vi "Test - Draw Teapot.vi"() -> ()   [LabVIEW 2022 SP3, in "Raster.lvlib"] (continued)
"y"=370.30228, "z"=0.9852259}, "UV"={"u"=0.0, "v"=0.0}, "Colour"=12517256}, "Vertex 3"={"Position"={"x"=479.53958, "y"=369.04208, "z"=0.98549163}, "UV"={"u"=0.0, "v"=0.0}, "Colour"=12517256}, "Alpha"=0.0, "Alpha Blending Enabled"=FALSE, "Colour"=11463293}, {"Vertex 1"={"Position"={"x"=221.22188, "y"=231.18608, "z"=0.9853604}, "UV"={"u"=0.0, "v"=0.0}, "Colour"=12517256}, "Vertex 2"={"Position"={"x"=225.54918, "y"=253.65358, "z"=0.9854739}, "UV"={"u"=0.0, "v"=0.0}, "Colour"=12517256}, "Vertex 3"={"Position"={"x"=257.52774, "y"=251.44232, "z"=0.9847784}, "UV"={"u"=0.0, "v"=0.0}, "Colour"=12517256}, "Alpha"=0.0, "Alpha Blending Enabled"=FALSE, "Colour"=9289317}, {"Vertex 1"={"Position"={"x"=479.53958, "y"=369.04208, "z"=0.98549163}, "UV"={"u"=0.0, "v"=0.0}, "Colour"=12517256}, "Vertex 2"={"Position"={"x"=484.57294, "y"=346.33105, "z"=0.98520327}, "UV"={"u"=0.0, "v"=0.0}, "Colour"=12517256}, "Vertex 3"={"Position"={"x"=444.34033, "y"=347.23126, "z"=0.9849148}, "UV"={"u"=0.0, "v"=0.0}, "Colour"=12517256}, "Alpha"=0.0, "Alpha Blending Enabled"=FALSE, "Colour"=11463293}, {"Vertex 1"={"Position"={"x"=486.9139, "y"=106.21548, "z"=0.98506916}, "UV"={"u"=0.0, "v"=0.0}, "Colour"=12517256}, "Vertex 2"={"Position"={"x"=481.5222, "y"=99.90905, "z"=0.985378}, "UV"={"u"=0.0, "v"=0.0}, "Colour"=12517256}, "Vertex 3"={"Position"={"x"=442.71094, "y"=96.16424, "z"=0.9851035}, "UV"={"u"=0.0, "v"=0.0}, "Colour"=12517256}, "Alpha"=0.0, "Alpha Blending Enabled"=FALSE, "Colour"=131841}, {"Vertex 1"={"Position"={"x"=315.42706, "y"=346.33105, "z"=0.98520327}, "UV"={"u"=0.0, "v"=0.0}, "Colour"=12517256}, "Vertex 2"={"Position"={"x"=310.53198, "y"=322.8849, "z"=0.98492277}, "UV"={"u"=0.0, "v"=0.0}, "Colour"=12517256}, "Vertex 3"={"Position"={"x"=274.2394, "y"=322.16803, "z"=0.9853966}, "UV"={"u"=0.0, "v"=0.0}, "Colour"=12517256}, "Alpha"=0.0, "Alpha Blending Enabled"=FALSE, "Colour"=11001975}, {"Vertex 1"={"Position"={"x"=277.72037, "y"=112.11777, "z"=0.98552537}, "UV"={"u"=0.0, "v"=0.0}, "Colour"=12517256}, "Vertex 2"={"Position"={"x"=270.06448, "y"=120.58319, "z"=0.98524225}, "UV"={"u"=0.0, "v"=0.0}, "Colour"=12517256}, "Vertex 3"={"Position"={"x"=307.46243, "y"=114.58211, "z"=0.98474693}, "UV"={"u"=0.0, "v"=0.0}, "Colour"=12517256}, "Alpha"=0.0, "Alpha Blending Enabled"=FALSE, "Colour"=131841}, {"Vertex 1"={"Position"={"x"=359.82788, "y"=91.52895, "z"=0.98539746}, "UV"={"u"=0.0, "v"=0.0}, "Colour"=12517256}, "Vertex 2"={"Position"={"x"=357.28906, "y"=96.16424, "z"=0.9851035}, "UV"={"u"=0.0, "v"=0.0}, "Colour"=12517256}, "Vertex 3"={"Position"={"x"=400.0, "y"=94.84046, "z"=0.9850064}, "UV"={"u"=0.0, "v"=0.0}, "Colour"=12517256}, "Alpha"=0.0, "Alpha Blending Enabled"=FALSE, "Colour"=131841}, {"Vertex 1"={"Position"={"x"=580.64856, "y"=168.66481, "z"=0.9853113}, "UV"={"u"=0.0, "v"=0.0}, "Colour"=12517256}, "Vertex 2"={"Position"={"x"=575.6004, "y"=152.34836, "z"=0.9854437}, "UV"={"u"=0.0, "v"=0.0}, "Colour"=12517256}, "Vertex 3"={"Position"={"x"=543.45624, "y"=145.25499, "z"=0.98474205}, "UV"={"u"=0.0, "v"=0.0}, "Colour"=12517256}, "Alpha"=0.0, "Alpha Blending Enabled"=FALSE, "Colour"=4413744}, {"Vertex 1"={"Position"={"x"=267.97037, "y"=298.8649, "z"=0.98516476}, "UV"={"u"=0.0, "v"=0.0}, "Colour"=12517256}, "Vertex 2"={"Position"={"x"=274.2394, "y"=322.16803, "z"=0.9853966}, "UV"={"u"=0.0, "v"=0.0}, "Colour"=12517256}, "Vertex 3"={"Position"={"x"=310.53198, "y"=322.8849, "z"=0.98492277}, "UV"={"u"=0.0, "v"=0.0}, "Colour"=12517256}, "Alpha"=0.0, "Alpha Blending Enabled"=FALSE, "Colour"=10804598}, {"Vertex 1"={"Position"={"x"=574.4508, "y"=253.65358, "z"=0.9854739}, "UV"={"u"=0.0, "v"=0.0}, "Colour"=12517256}, "Vertex 2"={"Position"={"x"=578.77814, "y"=231.18608, "z"=0.9853604}, "UV"={"u"=0.0, "v"=0.0}, "Colour"=12517256}, "Vertex 3"={"Position"={"x"=546.1793, "y"=227.81743, "z"=0.98464125}, "UV"={"u"=0.0, "v"=0.0}, "Colour"=12517256}, "Alpha"=0.0, "Alpha Blending Enabled"=FALSE, "Colour"=9289317}, {"Vertex 1"={"Position"={"x"=400.0, "y"=90.25612, "z"=0.985308}, "UV"={"u"=0.0, "v"=0.0}, "Colour"=12517256}, "Vertex 2"={"Position"={"x"=400.0, "y"=94.84046, "z"=0.9850064}, "UV"={"u"=0.0, "v"=0.0}, "Colour"=12517256}, "Vertex 3"={"Position"={"x"=442.71094, "y"=96.16424, "z"=0.9851035}, "UV"={"u"=0.0, "v"=0.0}, "Colour"=12517256}, "Alpha"=0.0, "Alpha Blending Enabled"=FALSE, "Colour"=131841}, {"Vertex 1"={"Position"={"x"=542.4723, "y"=251.44232, "z"=0.9847784}, "UV"={"u"=0.0, "v"=0.0}, "Colour"=12517256}, "Vertex 2"={"Position"={"x"=537.67664, "y"=275.21597, "z"=0.9849558}, "UV"={"u"=0.0, "v"=0.0}, "Colour"=12517256}, "Vertex 3"={"Position"={"x"=568.8375, "y"=276.3083, "z"=0.9856211}, "UV"={"u"=0.0, "v"=0.0}, "Colour"=12517256}, "Alpha"=0.0, "Alpha Blending Enabled"=FALSE, "Colour"=9750122}, {"Vertex 1"={"Position"={"x"=256.5438, "y"=145.25499, "z"=0.98474205}, "UV"={"u"=0.0, "v"=0.0}, "Colour"=12517256}, "Vertex 2"={"Position"={"x"=262.76135, "y"=131.49307, "z"=0.984972}, "UV"={"u"=0.0, "v"=0.0}, "Colour"=12517256}, "Vertex 3"={"Position"={"x"=231.67577, "y"=138.89714, "z"=0.98563457}, "UV"={"u"=0.0, "v"=0.0}, "Colour"=12517256}, "Alpha"=0.0, "Alpha Blending Enabled"=FALSE, "Colour"=2371610}, {"Vertex 1"={"Position"={"x"=358.34668, "y"=370.30228, "z"=0.9852259}, "UV"={"u"=0.0, "v"=0.0}, "Colour"=12517256}, "Vertex 2"={"Position"={"x"=355.65967, "y"=347.23126, "z"=0.9849148}, "UV"={"u"=0.0, "v"=0.0}, "Colour"=12517256}, "Vertex 3"={"Position"={"x"=315.42706, "y"=346.33105, "z"=0.98520327}, "UV"={"u"=0.0, "v"=0.0}, "Colour"=12517256}, "Alpha"=0.0, "Alpha Blending Enabled"=FALSE, "Colour"=11463293}, {"Vertex 1"={"Position"={"x"=307.46243, "y"=114.58211, "z"=0.98474693}, "UV"={"u"=0.0, "v"=0.0}, "Colour"=12517256}, "Vertex 2"={"Position"={"x"=313.0861, "y"=106.21548, "z"=0.98506916}, "UV"={"u"=0.0, "v"=0.0}, "Colour"=12517256}, "Vertex 3"={"Position"={"x"=277.72037, "y"=112.11777, "z"=0.98552537}, "UV"={"u"=0.0, "v"=0.0}, "Colour"=12517256}, "Alpha"=0.0, "Alpha Blending Enabled"=FALSE, "Colour"=131841}, {"Vertex 1"={"Position"={"x"=224.39961, "y"=152.34836, "z"=0.9854437}, "UV"={"u"=0.0, "v"=0.0}, "Colour"=12517256}, "Vertex 2"={"Position"={"x"=219.35144, "y"=168.66481, "z"=0.9853113}, "UV"={"u"=0.0, "v"=0.0}, "Colour"=12517256}, "Vertex 3"={"Position"={"x"=252.2155, "y"=162.16495, "z"=0.9845819}, "UV"={"u"=0.0, "v"=0.0}, "Colour"=12517256}, "Alpha"=0.0, "Alpha Blending Enabled"=FALSE, "Colour"=4413744}, {"Vertex 1"={"Position"={"x"=218.445, "y"=209.18083, "z"=0.98528755}, "UV"={"u"=0.0, "v"=0.0}, "Colour"=12517256}, "Vertex 2"={"Position"={"x"=221.22188, "y"=231.18608, "z"=0.9853604}, "UV"={"u"=0.0, "v"=0.0}, "Colour"=12517256}, "Vertex 3"={"Position"={"x"=253.82066, "y"=227.81743, "z"=0.98464125}, "UV"={"u"=0.0, "v"=0.0}, "Colour"=12517256}, "Alpha"=0.0, "Alpha Blending Enabled"=FALSE, "Colour"=8761951}, {"Vertex 1"={"Position"={"x"=355.65967, "y"=347.23126, "z"=0.9849148}, "UV"={"u"=0.0, "v"=0.0}, "Colour"=12517256}, "Vertex 2"={"Position"={"x"=358.34668, "y"=370.30228, "z"=0.9852259}, "UV"={"u"=0.0, "v"=0.0}, "Colour"=12517256}, "Vertex 3"={"Position"={"x"=400.0, "y"=370.74744, "z"=0.98513204}, "UV"={"u"=0.0, "v"=0.0}, "Colour"=12517256}, "Alpha"=0.0, "Alpha Blending Enabled"=FALSE, "Colour"=11660927}, {"Vertex 1"={"Position"={"x"=354.40778, "y"=102.34398, "z"=0.9847698}, "UV"={"u"=0.0, "v"=0.0}, "Colour"=12517256}, "Vertex 2"={"Position"={"x"=357.28906, "y"=96.16424, "z"=0.9851035}, "UV"={"u"=0.0, "v"=0.0}, "Colour"=12517256}, "Vertex 3"={"Position"={"x"=318.4778, "y"=99.90905, "z"=0.985378}, "UV"={"u"=0.0, "v"=0.0}, "Colour"=12517256}, "Alpha"=0.0, "Alpha Blending Enabled"=FALSE, "Colour"=131841}, {"Vertex 1"={"Position"={"x"=525.7606, "y"=322.16803, "z"=0.9853966}, "UV"={"u"=0.0, "v"=0.0}, "Colour"=12517256}, "Vertex 2"={"Position"={"x"=532.0296, "y"=298.8649, "z"=0.98516476}, "UV"={"u"=0.0, "v"=0.0}, "Colour"=12517256}, "Vertex 3"={"Position"={"x"=494.0796, "y"=298.8263, "z"=0.9846586}, "UV"={"u"=0.0, "v"=0.0}, "Colour"=12517256}, "Alpha"=0.0, "Alpha Blending Enabled"=FALSE, "Colour"=10804598}, {"Vertex 1"={"Position"={"x"=318.4778, "y"=99.90905, "z"=0.985378}, "UV"={"u"=0.0, "v"=0.0}, "Colour"=12517256}, "Vertex 2"={"Position"={"x"=313.0861, "y"=106.21548, "z"=0.98506916}, "UV"={"u"=0.0, "v"=0.0}, "Colour"=12517256}, "Vertex 3"={"Position"={"x"=354.40778, "y"=102.34398, "z"=0.9847698}, "UV"={"u"=0.0, "v"=0.0}, "Colour"=12517256}, "Alpha"=0.0, "Alpha Blending Enabled"=FALSE, "Colour"=131841}, {"Vertex 1"={"Position"={"x"=262.32336, "y"=275.21597, "z"=0.9849558}, "UV"={"u"=0.0, "v"=0.0}, "Colour"=12517256}, "Vertex 2"={"Position"={"x"=257.52774, "y"=251.44232, "z"=0.9847784}, "UV"={"u"=0.0, "v"=0.0}, "Colour"=12517256}, "Vertex 3"={"Position"={"x"=225.54918, "y"=253.65358, "z"=0.9854739}, "UV"={"u"=0.0, "v"=0.0}, "Colour"=12517256}, "Alpha"=0.0, "Alpha Blending Enabled"=FALSE, "Colour"=9750122}, {"Vertex 1"={"Position"={"x"=578.77814, "y"=231.18608, "z"=0.9853604}, "UV"={"u"=0.0, "v"=0.0}, "Colour"=12517256}, "Vertex 2"={"Position"={"x"=581.555, "y"=209.18083, "z"=0.98528755}, "UV"={"u"=0.0, "v"=0.0}, "Colour"=12517256}, "Vertex 3"={"Position"={"x"=548.5629, "y"=204.66248, "z"=0.9845531}, "UV"={"u"=0.0, "v"=0.0}, "Colour"=12517256}, "Alpha"=0.0, "Alpha Blending Enabled"=FALSE, "Colour"=8761951}, {"Vertex 1"={"Position"={"x"=400.0, "y"=347.54977, "z"=0.98481274}, "UV"={"u"=0.0, "v"=0.0}, "Colour"=12517256}, "Vertex 2"={"Position"={"x"=400.0, "y"=370.74744, "z"=0.98513204}, "UV"={"u"=0.0, "v"=0.0}, "Colour"=12517256}, "Vertex 3"={"Position"={"x"=441.6533, "y"=370.30228, "z"=0.9852259}, "UV"={"u"=0.0, "v"=0.0}, "Colour"=12517256}, "Alpha"=0.0, "Alpha Blending Enabled"=FALSE, "Colour"=11660927}, {"Vertex 1"={"Position"={"x"=537.23865, "y"=131.49307, "z"=0.984972}, "UV"={"u"=0.0, "v"=0.0}, "Colour"=12517256}, "Vertex 2"={"Position"={"x"=543.45624, "y"=145.25499, "z"=0.98474205}, "UV"={"u"=0.0, "v"=0.0}, "Colour"=12517256}, "Vertex 3"={"Position"={"x"=575.6004, "y"=152.34836, "z"=0.9854437}, "UV"={"u"=0.0, "v"=0.0}, "Colour"=12517256}, "Alpha"=0.0, "Alpha Blending Enabled"=FALSE, "Colour"=2371610}, {"Vertex 1"={"Position"={"x"=582.5317, "y"=187.944, "z"=0.9852619}, "UV"={"u"=0.0, "v"=0.0}, "Colour"=12517256}, "Vertex 2"={"Position"={"x"=580.64856, "y"=168.66481, "z"=0.9853113}, "UV"={"u"=0.0, "v"=0.0}, "Colour"=12517256}, "Vertex 3"={"Position"={"x"=547.78455, "y"=162.16495, "z"=0.9845819}, "UV"={"u"=0.0, "v"=0.0}, "Colour"=12517256}, "Alpha"=0.0, "Alpha Blending Enabled"=FALSE, "Colour"=6522183}, {"Vertex 1"={"Position"={"x"=217.4683, "y"=187.944, "z"=0.9852619}, "UV"={"u"=0.0, "v"=0.0}, "Colour"=12517256}, "Vertex 2"={"Position"={"x"=218.445, "y"=209.18083, "z"=0.98528755}, "UV"={"u"=0.0, "v"=0.0}, "Colour"=12517256}, "Vertex 3"={"Position"={"x"=251.43709, "y"=204.66248, "z"=0.9845531}, "UV"={"u"=0.0, "v"=0.0}, "Colour"=12517256}, "Alpha"=0.0, "Alpha Blending Enabled"=FALSE, "Colour"=7971671}, {"Vertex 1"={"Position"={"x"=219.35144, "y"=168.66481, "z"=0.9853113}, "UV"={"u"=0.0, "v"=0.0}, "Colour"=12517256}, "Vertex 2"={"Position"={"x"=217.4683, "y"=187.944, "z"=0.9852619}, "UV"={"u"=0.0, "v"=0.0}, "Colour"=12517256}, "Vertex 3"={"Position"={"x"=250.598, "y"=182.33759, "z"=0.9845221}, "UV"={"u"=0.0, "v"=0.0}, "Colour"=12517256}, "Alpha"=0.0, "Alpha Blending Enabled"=FALSE, "Colour"=6522183}, {"Vertex 1"={"Position"={"x"=581.555, "y"=209.18083, "z"=0.98528755}, "UV"={"u"=0.0, "v"=0.0}, "Colour"=12517256}, "Vertex 2"={"Position"={"x"=582.5317, "y"=187.944, "z"=0.9852619}, "UV"={"u"=0.0, "v"=0.0}, "Colour"=12517256}, "Vertex 3"={"Position"={"x"=549.402, "y"=182.33759, "z"=0.9845221}, "UV"={"u"=0.0, "v"=0.0}, "Colour"=12517256}, "Alpha"=0.0, "Alpha Blending Enabled"=FALSE, "Colour"=7971671}, {"Vertex 1"={"Position"={"x"=486.9139, "y"=106.21548, "z"=0.98506916}, "UV"={"u"=0.0, "v"=0.0}, "Colour"=12517256}, "Vertex 2"={"Position"={"x"=492.5376, "y"=114.58211, "z"=0.98474693}, "UV"={"u"=0.0, "v"=0.0}, "Colour"=12517256}, "Vertex 3"={"Position"={"x"=529.9355, "y"=120.58319, "z"=0.98524225}, "UV"={"u"=0.0, "v"=0.0}, "Colour"=12517256}, "Alpha"=0.0, "Alpha Blending Enabled"=FALSE, "Colour"=131841}, {"Vertex 1"={"Position"={"x"=310.53198, "y"=322.8849, "z"=0.98492277}, "UV"={"u"=0.0, "v"=0.0}, "Colour"=12517256}, "Vertex 2"={"Position"={"x"=315.42706, "y"=346.33105, "z"=0.98520327}, "UV"={"u"=0.0, "v"=0.0}, "Colour"=12517256}, "Vertex 3"={"Position"={"x"=355.65967, "y"=347.23126, "z"=0.9849148}, "UV"={"u"=0.0, "v"=0.0}, "Colour"=12517256}, "Alpha"=0.0, "Alpha Blending Enabled"=FALSE, "Colour"=11397244}, {"Vertex 1"={"Position"={"x"=494.0796, "y"=298.8263, "z"=0.9846586}, "UV"={"u"=0.0, "v"=0.0}, "Colour"=12517256}, "Vertex 2"={"Position"={"x"=489.46802, "y"=322.8849, "z"=0.98492277}, "UV"={"u"=0.0, "v"=0.0}, "Colour"=12517256}, "Vertex 3"={"Position"={"x"=525.7606, "y"=322.16803, "z"=0.9853966}, "UV"={"u"=0.0, "v"=0.0}, "Colour"=12517256}, "Alpha"=0.0, "Alpha Blending Enabled"=FALSE, "Colour"=10804598}, {"Vertex 1"={"Position"={"x"=537.23865, "y"=131.49307, "z"=0.984972}, "UV"={"u"=0.0, "v"=0.0}, "Colour"=12517256}, "Vertex 2"={"Position"={"x"=529.9355, "y"=120.58319, "z"=0.98524225}, "UV"={"u"=0.0, "v"=0.0}, "Colour"=12517256}, "Vertex 3"={"Position"={"x"=492.5376, "y"=114.58211, "z"=0.98474693}, "UV"={"u"=0.0, "v"=0.0}, "Colour"=12517256}, "Alpha"=0.0, "Alpha Blending Enabled"=FALSE, "Colour"=1251597}, {"Vertex 1"={"Position"={"x"=441.6533, "y"=370.30228, "z"=0.9852259}, "UV"={"u"=0.0, "v"=0.0}, "Colour"=12517256}, "Vertex 2"={"Position"={"x"=444.34033, "y"=347.23126, "z"=0.9849148}, "UV"={"u"=0.0, "v"=0.0}, "Colour"=12517256}, "Vertex 3"={"Position"={"x"=400.0, "y"=347.54977, "z"=0.98481274}, "UV"={"u"=0.0, "v"=0.0}, "Colour"=12517256}, "Alpha"=0.0, "Alpha Blending Enabled"=FALSE, "Colour"=11660927}, {"Vertex 1"={"Position"={"x"=442.71094, "y"=96.16424, "z"=0.9851035}, "UV"={"u"=0.0, "v"=0.0}, "Colour"=12517256}, "Vertex 2"={"Position"={"x"=445.59222, "y"=102.34398, "z"=0.9847698}, "UV"={"u"=0.0, "v"=0.0}, "Colour"=12517256}, "Vertex 3"={"Position"={"x"=486.9139, "y"=106.21548, "z"=0.98506916}, "UV"={"u"=0.0, "v"=0.0}, "Colour"=12517256}, "Alpha"=0.0, "Alpha Blending Enabled"=FALSE, "Colour"=131841}, {"Vertex 1"={"Position"={"x"=546.1793, "y"=227.81743, "z"=0.98464125}, "UV"={"u"=0.0, "v"=0.0}, "Colour"=12517256}, "Vertex 2"={"Position"={"x"=542.4723, "y"=251.44232, "z"=0.9847784}, "UV"={"u"=0.0, "v"=0.0}, "Colour"=12517256}, "Vertex 3"={"Position"={"x"=574.4508, "y"=253.65358, "z"=0.9854739}, "UV"={"u"=0.0, "v"=0.0}, "Colour"=12517256}, "Alpha"=0.0, "Alpha Blending Enabled"=FALSE, "Colour"=9289317}, {"Vertex 1"={"Position"={"x"=445.59222, "y"=102.34398, "z"=0.9847698}, "UV"={"u"=0.0, "v"=0.0}, "Colour"=12517256}, "Vertex 2"={"Position"={"x"=442.71094, "y"=96.16424, "z"=0.9851035}, "UV"={"u"=0.0, "v"=0.0}, "Colour"=12517256}, "Vertex 3"={"Position"={"x"=400.0, "y"=94.84046, "z"=0.9850064}, "UV"={"u"=0.0, "v"=0.0}, "Colour"=12517256}, "Alpha"=0.0, "Alpha Blending Enabled"=FALSE, "Colour"=131841}, {"Vertex 1"={"Position"={"x"=400.0, "y"=370.74744, "z"=0.98513204}, "UV"={"u"=0.0, "v"=0.0}, "Colour"=12517256}, "Vertex 2"={"Position"={"x"=400.0, "y"=347.54977, "z"=0.98481274}, "UV"={"u"=0.0, "v"=0.0}, "Colour"=12517256}, "Vertex 3"={"Position"={"x"=355.65967, "y"=347.23126, "z"=0.9849148}, "UV"={"u"=0.0, "v"=0.0}, "Colour"=12517256}, "Alpha"=0.0, "Alpha Blending Enabled"=FALSE, "Colour"=11660927}, {"Vertex 1"={"Position"={"x"=257.52774, "y"=251.44232, "z"=0.9847784}, "UV"={"u"=0.0, "v"=0.0}, "Colour"=12517256}, "Vertex 2"={"Position"={"x"=253.82066, "y"=227.81743, "z"=0.98464125}, "UV"={"u"=0.0, "v"=0.0}, "Colour"=12517256}, "Vertex 3"={"Position"={"x"=221.22188, "y"=231.18608, "z"=0.9853604}, "UV"={"u"=0.0, "v"=0.0}, "Colour"=12517256}, "Alpha"=0.0, "Alpha Blending Enabled"=FALSE, "Colour"=9289317}, {"Vertex 1"={"Position"={"x"=262.32336, "y"=275.21597, "z"=0.9849558}, "UV"={"u"=0.0, "v"=0.0}, "Colour"=12517256}, "Vertex 2"={"Position"={"x"=267.97037, "y"=298.8649, "z"=0.98516476}, "UV"={"u"=0.0, "v"=0.0}, "Colour"=12517256}, "Vertex 3"={"Position"={"x"=305.9204, "y"=298.8263, "z"=0.9846586}, "UV"={"u"=0.0, "v"=0.0}, "Colour"=12517256}, "Alpha"=0.0, "Alpha Blending Enabled"=FALSE, "Colour"=10606707}, {"Vertex 1"={"Position"={"x"=400.0, "y"=100.973206, "z"=0.98466384}, "UV"={"u"=0.0, "v"=0.0}, "Colour"=12517256}, "Vertex 2"={"Position"={"x"=400.0, "y"=94.84046, "z"=0.9850064}, "UV"={"u"=0.0, "v"=0.0}, "Colour"=12517256}, "Vertex 3"={"Position"={"x"=357.28906, "y"=96.16424, "z"=0.9851035}, "UV"={"u"=0.0, "v"=0.0}, "Colour"=12517256}, "Alpha"=0.0, "Alpha Blending Enabled"=FALSE, "Colour"=131841}, {"Vertex 1"={"Position"={"x"=252.2155, "y"=162.16495, "z"=0.9845819}, "UV"={"u"=0.0, "v"=0.0}, "Colour"=12517256}, "Vertex 2"={"Position"={"x"=256.5438, "y"=145.25499, "z"=0.98474205}, "UV"={"u"=0.0, "v"=0.0}, "Colour"=12517256}, "Vertex 3"={"Position"={"x"=224.39961, "y"=152.34836, "z"=0.9854437}, "UV"={"u"=0.0, "v"=0.0}, "Colour"=12517256}, "Alpha"=0.0, "Alpha Blending Enabled"=FALSE, "Colour"=4413744}, {"Vertex 1"={"Position"={"x"=310.53198, "y"=322.8849, "z"=0.98492277}, "UV"={"u"=0.0, "v"=0.0}, "Colour"=12517256}, "Vertex 2"={"Position"={"x"=305.9204, "y"=298.8263, "z"=0.9846586}, "UV"={"u"=0.0, "v"=0.0}, "Colour"=12517256}, "Vertex 3"={"Position"={"x"=267.97037, "y"=298.8649, "z"=0.98516476}, "UV"={"u"=0.0, "v"=0.0}, "Colour"=12517256}, "Alpha"=0.0, "Alpha Blending Enabled"=FALSE, "Colour"=10804598}, {"Vertex 1"={"Position"={"x"=484.57294, "y"=346.33105, "z"=0.98520327}, "UV"={"u"=0.0, "v"=0.0}, "Colour"=12517256}, "Vertex 2"={"Position"={"x"=489.46802, "y"=322.8849, "z"=0.98492277}, "UV"={"u"=0.0, "v"=0.0}, "Colour"=12517256}, "Vertex 3"={"Position"={"x"=446.95963, "y"=323.3558, "z"=0.9846115}, "UV"={"u"=0.0, "v"=0.0}, "Colour"=12517256}, "Alpha"=0.0, "Alpha Blending Enabled"=FALSE, "Colour"=11397244}, {"Vertex 1"={"Position"={"x"=446.95963, "y"=323.3558, "z"=0.9846115}, "UV"={"u"=0.0, "v"=0.0}, "Colour"=12517256}, "Vertex 2"={"Position"={"x"=444.34033, "y"=347.23126, "z"=0.9849148}, "UV"={"u"=0.0, "v"=0.0}, "Colour"=12517256}, "Vertex 3"={"Position"={"x"=484.57294, "y"=346.33105, "z"=0.98520327}, "UV"={"u"=0.0, "v"=0.0}, "Colour"=12517256}, "Alpha"=0.0, "Alpha Blending Enabled"=FALSE, "Colour"=11397244}, {"Vertex 1"={"Position"={"x"=270.06448, "y"=120.58319, "z"=0.98524225}, "UV"={"u"=0.0, "v"=0.0}, "Colour"=12517256}, "Vertex 2"={"Position"={"x"=262.76135, "y"=131.49307, "z"=0.984972}, "UV"={"u"=0.0, "v"=0.0}, "Colour"=12517256}, "Vertex 3"={"Position"={"x"=302.07715, "y"=125.52894, "z"=0.98443836}, "UV"={"u"=0.0, "v"=0.0}, "Colour"=12517256}, "Alpha"=0.0, "Alpha Blending Enabled"=FALSE, "Colour"=1251597}, {"Vertex 1"={"Position"={"x"=543.45624, "y"=145.25499, "z"=0.98474205}, "UV"={"u"=0.0, "v"=0.0}, "Colour"=12517256}, "Vertex 2"={"Position"={"x"=547.78455, "y"=162.16495, "z"=0.9845819}, "UV"={"u"=0.0, "v"=0.0}, "Colour"=12517256}, "Vertex 3"={"Position"={"x"=580.64856, "y"=168.66481, "z"=0.9853113}, "UV"={"u"=0.0, "v"=0.0}, "Colour"=12517256}, "Alpha"=0.0, "Alpha Blending Enabled"=FALSE, "Colour"=4413744}, {"Vertex 1"={"Position"={"x"=492.5376, "y"=114.58211, "z"=0.98474693}, "UV"={"u"=0.0, "v"=0.0}, "Colour"=12517256}, "Vertex 2"={"Position"={"x"=486.9139, "y"=106.21548, "z"=0.98506916}, "UV"={"u"=0.0, "v"=0.0}, "Colour"=12517256}, "Vertex 3"={"Position"={"x"=445.59222, "y"=102.34398, "z"=0.9847698}, "UV"={"u"=0.0, "v"=0.0}, "Colour"=12517256}, "Alpha"=0.0, "Alpha Blending Enabled"=FALSE, "Colour"=197890}, {"Vertex 1"={"Position"={"x"=548.5629, "y"=204.66248, "z"=0.9845531}, "UV"={"u"=0.0, "v"=0.0}, "Colour"=12517256}, "Vertex 2"={"Position"={"x"=546.1793, "y"=227.81743, "z"=0.98464125}, "UV"={"u"=0.0, "v"=0.0}, "Colour"=12517256}, "Vertex 3"={"Position"={"x"=578.77814, "y"=231.18608, "z"=0.9853604}, "UV"={"u"=0.0, "v"=0.0}, "Colour"=12517256}, "Alpha"=0.0, "Alpha Blending Enabled"=FALSE, "Colour"=8761951}, {"Vertex 1"={"Position"={"x"=532.0296, "y"=298.8649, "z"=0.98516476}, "UV"={"u"=0.0, "v"=0.0}, "Colour"=12517256}, "Vertex 2"={"Position"={"x"=537.67664, "y"=275.21597, "z"=0.9849558}, "UV"={"u"=0.0, "v"=0.0}, "Colour"=12517256}, "Vertex 3"={"Position"={"x"=498.2464, "y"=274.33585, "z"=0.9844198}, "UV"={"u"=0.0, "v"=0.0}, "Colour"=12517256}, "Alpha"=0.0, "Alpha Blending Enabled"=FALSE, "Colour"=10606707}, {"Vertex 1"={"Position"={"x"=357.28906, "y"=96.16424, "z"=0.9851035}, "UV"={"u"=0.0, "v"=0.0}, "Colour"=12517256}, "Vertex 2"={"Position"={"x"=354.40778, "y"=102.34398, "z"=0.9847698}, "UV"={"u"=0.0, "v"=0.0}, "Colour"=12517256}, "Vertex 3"={"Position"={"x"=400.0, "y"=100.973206, "z"=0.98466384}, "UV"={"u"=0.0, "v"=0.0}, "Colour"=12517256}, "Alpha"=0.0, "Alpha Blending Enabled"=FALSE, "Colour"=131841}, {"Vertex 1"={"Position"={"x"=253.82066, "y"=227.81743, "z"=0.98464125}, "UV"={"u"=0.0, "v"=0.0}, "Colour"=12517256}, "Vertex 2"={"Position"={"x"=251.43709, "y"=204.66248, "z"=0.9845531}, "UV"={"u"=0.0, "v"=0.0}, "Colour"=12517256}, "Vertex 3"={"Position"={"x"=218.445, "y"=209.18083, "z"=0.98528755}, "UV"={"u"=0.0, "v"=0.0}, "Colour"=12517256}, "Alpha"=0.0, "Alpha Blending Enabled"=FALSE, "Colour"=8761951}, {"Vertex 1"={"Position"={"x"=355.65967, "y"=347.23126, "z"=0.9849148}, "UV"={"u"=0.0, "v"=0.0}, "Colour"=12517256}, "Vertex 2"={"Position"={"x"=353.04034, "y"=323.3558, "z"=0.9846115}, "UV"={"u"=0.0, "v"=0.0}, "Colour"=12517256}, "Vertex 3"={"Position"={"x"=310.53198, "y"=322.8849, "z"=0.98492277}, "UV"={"u"=0.0, "v"=0.0}, "Colour"=12517256}, "Alpha"=0.0, "Alpha Blending Enabled"=FALSE, "Colour"=11397244}, {"Vertex 1"={"Position"={"x"=400.0, "y"=94.84046, "z"=0.9850064}, "UV"={"u"=0.0, "v"=0.0}, "Colour"=12517256}, "Vertex 2"={"Position"={"x"=400.0, "y"=100.973206, "z"=0.98466384}, "UV"={"u"=0.0, "v"=0.0}, "Colour"=12517256}, "Vertex 3"={"Position"={"x"=445.59222, "y"=102.34398, "z"=0.9847698}, "UV"={"u"=0.0, "v"=0.0}, "Colour"=12517256}, "Alpha"=0.0, "Alpha Blending Enabled"=FALSE, "Colour"=131841}, {"Vertex 1"={"Position"={"x"=302.07715, "y"=125.52894, "z"=0.98443836}, "UV"={"u"=0.0, "v"=0.0}, "Colour"=12517256}, "Vertex 2"={"Position"={"x"=307.46243, "y"=114.58211, "z"=0.98474693}, "UV"={"u"=0.0, "v"=0.0}, "Colour"=12517256}, "Vertex 3"={"Position"={"x"=270.06448, "y"=120.58319, "z"=0.98524225}, "UV"={"u"=0.0, "v"=0.0}, "Colour"=12517256}, "Alpha"=0.0, "Alpha Blending Enabled"=FALSE, "Colour"=1251597}, {"Vertex 1"={"Position"={"x"=250.598, "y"=182.33759, "z"=0.9845221}, "UV"={"u"=0.0, "v"=0.0}, "Colour"=12517256}, "Vertex 2"={"Position"={"x"=252.2155, "y"=162.16495, "z"=0.9845819}, "UV"={"u"=0.0, "v"=0.0}, "Colour"=12517256}, "Vertex 3"={"Position"={"x"=219.35144, "y"=168.66481, "z"=0.9853113}, "UV"={"u"=0.0, "v"=0.0}, "Colour"=12517256}, "Alpha"=0.0, "Alpha Blending Enabled"=FALSE, "Colour"=6522183}, {"Vertex 1"={"Position"={"x"=547.78455, "y"=162.16495, "z"=0.9845819}, "UV"={"u"=0.0, "v"=0.0}, "Colour"=12517256}, "Vertex 2"={"Position"={"x"=549.402, "y"=182.33759, "z"=0.9845221}, "UV"={"u"=0.0, "v"=0.0}, "Colour"=12517256}, "Vertex 3"={"Position"={"x"=582.5317, "y"=187.944, "z"=0.9852619}, "UV"={"u"=0.0, "v"=0.0}, "Colour"=12517256}, "Alpha"=0.0, "Alpha Blending Enabled"=FALSE, "Colour"=6522183}, {"Vertex 1"={"Position"={"x"=549.402, "y"=182.33759, "z"=0.9845221}, "UV"={"u"=0.0, "v"=0.0}, "Colour"=12517256}, "Vertex 2"={"Position"={"x"=548.5629, "y"=204.66248, "z"=0.9845531}, "UV"={"u"=0.0, "v"=0.0}, "Colour"=12517256}, "Vertex 3"={"Position"={"x"=581.555, "y"=209.18083, "z"=0.98528755}, "UV"={"u"=0.0, "v"=0.0}, "Colour"=12517256}, "Alpha"=0.0, "Alpha Blending Enabled"=FALSE, "Colour"=7971671}, {"Vertex 1"={"Position"={"x"=353.04034, "y"=323.3558, "z"=0.9846115}, "UV"={"u"=0.0, "v"=0.0}, "Colour"=12517256}, "Vertex 2"={"Position"={"x"=355.65967, "y"=347.23126, "z"=0.9849148}, "UV"={"u"=0.0, "v"=0.0}, "Colour"=12517256}, "Vertex 3"={"Position"={"x"=400.0, "y"=347.54977, "z"=0.98481274}, "UV"={"u"=0.0, "v"=0.0}, "Colour"=12517256}, "Alpha"=0.0, "Alpha Blending Enabled"=FALSE, "Colour"=11594878}, {"Vertex 1"={"Position"={"x"=251.43709, "y"=204.66248, "z"=0.9845531}, "UV"={"u"=0.0, "v"=0.0}, "Colour"=12517256}, "Vertex 2"={"Position"={"x"=250.598, "y"=182.33759, "z"=0.9845221}, "UV"={"u"=0.0, "v"=0.0}, "Colour"=12517256}, "Vertex 3"={"Position"={"x"=217.4683, "y"=187.944, "z"=0.9852619}, "UV"={"u"=0.0, "v"=0.0}, "Colour"=12517256}, "Alpha"=0.0, "Alpha Blending Enabled"=FALSE, "Colour"=7971671}, {"Vertex 1"={"Position"={"x"=351.39496, "y"=110.63302, "z"=0.984421}, "UV"={"u"=0.0, "v"=0.0}, "Colour"=12517256}, "Vertex 2"={"Position"={"x"=354.40778, "y"=102.34398, "z"=0.9847698}, "UV"={"u"=0.0, "v"=0.0}, "Colour"=12517256}, "Vertex 3"={"Position"={"x"=313.0861, "y"=106.21548, "z"=0.98506916}, "UV"={"u"=0.0, "v"=0.0}, "Colour"=12517256}, "Alpha"=0.0, "Alpha Blending Enabled"=FALSE, "Colour"=197890}, {"Vertex 1"={"Position"={"x"=498.2464, "y"=274.33585, "z"=0.9844198}, "UV"={"u"=0.0, "v"=0.0}, "Colour"=12517256}, "Vertex 2"={"Position"={"x"=494.0796, "y"=298.8263, "z"=0.9846586}, "UV"={"u"=0.0, "v"=0.0}, "Colour"=12517256}, "Vertex 3"={"Position"={"x"=532.0296, "y"=298.8649, "z"=0.98516476}, "UV"={"u"=0.0, "v"=0.0}, "Colour"=12517256}, "Alpha"=0.0, "Alpha Blending Enabled"=FALSE, "Colour"=10606707}, {"Vertex 1"={"Position"={"x"=313.0861, "y"=106.21548, "z"=0.98506916}, "UV"={"u"=0.0, "v"=0.0}, "Colour"=12517256}, "Vertex 2"={"Position"={"x"=307.46243, "y"=114.58211, "z"=0.98474693}, "UV"={"u"=0.0, "v"=0.0}, "Colour"=12517256}, "Vertex 3"={"Position"={"x"=351.39496, "y"=110.63302, "z"=0.984421}, "UV"={"u"=0.0, "v"=0.0}, "Colour"=12517256}, "Alpha"=0.0, "Alpha Blending Enabled"=FALSE, "Colour"=197890}, {"Vertex 1"={"Position"={"x"=400.0, "y"=323.52267, "z"=0.9845012}, "UV"={"u"=0.0, "v"=0.0}, "Colour"=12517256}, "Vertex 2"={"Position"={"x"=400.0, "y"=347.54977, "z"=0.98481274}, "UV"={"u"=0.0, "v"=0.0}, "Colour"=12517256}, "Vertex 3"={"Position"={"x"=444.34033, "y"=347.23126, "z"=0.9849148}, "UV"={"u"=0.0, "v"=0.0}, "Colour"=12517256}, "Alpha"=0.0, "Alpha Blending Enabled"=FALSE, "Colour"=11594878}, {"Vertex 1"={"Position"={"x"=305.9204, "y"=298.8263, "z"=0.9846586}, "UV"={"u"=0.0, "v"=0.0}, "Colour"=12517256}, "Vertex 2"={"Position"={"x"=310.53198, "y"=322.8849, "z"=0.98492277}, "UV"={"u"=0.0, "v"=0.0}, "Colour"=12517256}, "Vertex 3"={"Position"={"x"=353.04034, "y"=323.3558, "z"=0.9846115}, "UV"={"u"=0.0, "v"=0.0}, "Colour"=12517256}, "Alpha"=0.0, "Alpha Blending Enabled"=FALSE, "Colour"=11199866}, {"Vertex 1"={"Position"={"x"=492.5376, "y"=114.58211, "z"=0.98474693}, "UV"={"u"=0.0, "v"=0.0}, "Colour"=12517256}, "Vertex 2"={"Position"={"x"=497.92285, "y"=125.52894, "z"=0.98443836}, "UV"={"u"=0.0, "v"=0.0}, "Colour"=12517256}, "Vertex 3"={"Position"={"x"=537.23865, "y"=131.49307, "z"=0.984972}, "UV"={"u"=0.0, "v"=0.0}, "Colour"=12517256}, "Alpha"=0.0, "Alpha Blending Enabled"=FALSE, "Colour"=1251597}, {"Vertex 1"={"Position"={"x"=257.52774, "y"=251.44232, "z"=0.9847784}, "UV"={"u"=0.0, "v"=0.0}, "Colour"=12517256}, "Vertex 2"={"Position"={"x"=262.32336, "y"=275.21597, "z"=0.9849558}, "UV"={"u"=0.0, "v"=0.0}, "Colour"=12517256}, "Vertex 3"={"Position"={"x"=301.7536, "y"=274.33585, "z"=0.9844198}, "UV"={"u"=0.0, "v"=0.0}, "Colour"=12517256}, "Alpha"=0.0, "Alpha Blending Enabled"=FALSE, "Colour"=10343024}, {"Vertex 1"={"Position"={"x"=543.45624, "y"=145.25499, "z"=0.98474205}, "UV"={"u"=0.0, "v"=0.0}, "Colour"=12517256}, "Vertex 2"={"Position"={"x"=537.23865, "y"=131.49307, "z"=0.984972}, "UV"={"u"=0.0, "v"=0.0}, "Colour"=12517256}, "Vertex 3"={"Position"={"x"=497.92285, "y"=125.52894, "z"=0.98443836}, "UV"={"u"=0.0, "v"=0.0}, "Colour"=12517256}, "Alpha"=0.0, "Alpha Blending Enabled"=FALSE, "Colour"=2964512}, {"Vertex 1"={"Position"={"x"=305.9204, "y"=298.8263, "z"=0.9846586}, "UV"={"u"=0.0, "v"=0.0}, "Colour"=12517256}, "Vertex 2"={"Position"={"x"=301.7536, "y"=274.33585, "z"=0.9844198}, "UV"={"u"=0.0, "v"=0.0}, "Colour"=12517256}, "Vertex 3"={"Position"={"x"=262.32336, "y"=275.21597, "z"=0.9849558}, "UV"={"u"=0.0, "v"=0.0}, "Colour"=12517256}, "Alpha"=0.0, "Alpha Blending Enabled"=FALSE, "Colour"=10606707}, {"Vertex 1"={"Position"={"x"=444.34033, "y"=347.23126, "z"=0.9849148}, "UV"={"u"=0.0, "v"=0.0}, "Colour"=12517256}, "Vertex 2"={"Position"={"x"=446.95963, "y"=323.3558, "z"=0.9846115}, "UV"={"u"=0.0, "v"=0.0}, "Colour"=12517256}, "Vertex 3"={"Position"={"x"=400.0, "y"=323.52267, "z"=0.9845012}, "UV"={"u"=0.0, "v"=0.0}, "Colour"=12517256}, "Alpha"=0.0, "Alpha Blending Enabled"=FALSE, "Colour"=11594878}, {"Vertex 1"={"Position"={"x"=537.67664, "y"=275.21597, "z"=0.9849558}, "UV"={"u"=0.0, "v"=0.0}, "Colour"=12517256}, "Vertex 2"={"Position"={"x"=542.4723, "y"=251.44232, "z"=0.9847784}, "UV"={"u"=0.0, "v"=0.0}, "Colour"=12517256}, "Vertex 3"={"Position"={"x"=501.79443, "y"=249.65573, "z"=0.9842166}, "UV"={"u"=0.0, "v"=0.0}, "Colour"=12517256}, "Alpha"=0.0, "Alpha Blending Enabled"=FALSE, "Colour"=10343024}, {"Vertex 1"={"Position"={"x"=445.59222, "y"=102.34398, "z"=0.9847698}, "UV"={"u"=0.0, "v"=0.0}, "Colour"=12517256}, "Vertex 2"={"Position"={"x"=448.60507, "y"=110.63302, "z"=0.984421}, "UV"={"u"=0.0, "v"=0.0}, "Colour"=12517256}, "Vertex 3"={"Position"={"x"=492.5376, "y"=114.58211, "z"=0.98474693}, "UV"={"u"=0.0, "v"=0.0}, "Colour"=12517256}, "Alpha"=0.0, "Alpha Blending Enabled"=FALSE, "Colour"=197890}, {"Vertex 1"={"Position"={"x"=400.0, "y"=347.54977, "z"=0.98481274}, "UV"={"u"=0.0, "v"=0.0}, "Colour"=12517256}, "Vertex 2"={"Position"={"x"=400.0, "y"=323.52267, "z"=0.9845012}, "UV"={"u"=0.0, "v"=0.0}, "Colour"=12517256}, "Vertex 3"={"Position"={"x"=353.04034, "y"=323.3558, "z"=0.9846115}, "UV"={"u"=0.0, "v"=0.0}, "Colour"=12517256}, "Alpha"=0.0, "Alpha Blending Enabled"=FALSE, "Colour"=11594878}, {"Vertex 1"={"Position"={"x"=489.46802, "y"=322.8849, "z"=0.98492277}, "UV"={"u"=0.0, "v"=0.0}, "Colour"=12517256}, "Vertex 2"={"Position"={"x"=494.0796, "y"=298.8263, "z"=0.9846586}, "UV"={"u"=0.0, "v"=0.0}, "Colour"=12517256}, "Vertex 3"={"Position"={"x"=449.43246, "y"=298.80087, "z"=0.9843252}, "UV"={"u"=0.0, "v"=0.0}, "Colour"=12517256}, "Alpha"=0.0, "Alpha Blending Enabled"=FALSE, "Colour"=11199866}, {"Vertex 1"={"Position"={"x"=262.76135, "y"=131.49307, "z"=0.984972}, "UV"={"u"=0.0, "v"=0.0}, "Colour"=12517256}, "Vertex 2"={"Position"={"x"=256.5438, "y"=145.25499, "z"=0.98474205}, "UV"={"u"=0.0, "v"=0.0}, "Colour"=12517256}, "Vertex 3"={"Position"={"x"=297.47644, "y"=139.52065, "z"=0.9841747}, "UV"={"u"=0.0, "v"=0.0}, "Colour"=12517256}, "Alpha"=0.0, "Alpha Blending Enabled"=FALSE, "Colour"=2964512}, {"Vertex 1"={"Position"={"x"=449.43246, "y"=298.80087, "z"=0.9843252}, "UV"={"u"=0.0, "v"=0.0}, "Colour"=12517256}, "Vertex 2"={"Position"={"x"=446.95963, "y"=323.3558, "z"=0.9846115}, "UV"={"u"=0.0, "v"=0.0}, "Colour"=12517256}, "Vertex 3"={"Position"={"x"=489.46802, "y"=322.8849, "z"=0.98492277}, "UV"={"u"=0.0, "v"=0.0}, "Colour"=12517256}, "Alpha"=0.0, "Alpha Blending Enabled"=FALSE, "Colour"=11199866}, {"Vertex 1"={"Position"={"x"=448.60507, "y"=110.63302, "z"=0.984421}, "UV"={"u"=0.0, "v"=0.0}, "Colour"=12517256}, "Vertex 2"={"Position"={"x"=445.59222, "y"=102.34398, "z"=0.9847698}, "UV"={"u"=0.0, "v"=0.0}, "Colour"=12517256}, "Vertex 3"={"Position"={"x"=400.0, "y"=100.973206, "z"=0.98466384}, "UV"={"u"=0.0, "v"=0.0}, "Colour"=12517256}, "Alpha"=0.0, "Alpha Blending Enabled"=FALSE, "Colour"=395268}, {"Vertex 1"={"Position"={"x"=400.0, "y"=109.232285, "z"=0.9843054}, "UV"={"u"=0.0, "v"=0.0}, "Colour"=12517256}, "Vertex 2"={"Position"={"x"=400.0, "y"=100.973206, "z"=0.98466384}, "UV"={"u"=0.0, "v"=0.0}, "Colour"=12517256}, "Vertex 3"={"Position"={"x"=354.40778, "y"=102.34398, "z"=0.9847698}, "UV"={"u"=0.0, "v"=0.0}, "Colour"=12517256}, "Alpha"=0.0, "Alpha Blending Enabled"=FALSE, "Colour"=395268}, {"Vertex 1"={"Position"={"x"=253.82066, "y"=227.81743, "z"=0.98464125}, "UV"={"u"=0.0, "v"=0.0}, "Colour"=12517256}, "Vertex 2"={"Position"={"x"=257.52774, "y"=251.44232, "z"=0.9847784}, "UV"={"u"=0.0, "v"=0.0}, "Colour"=12517256}, "Vertex 3"={"Position"={"x"=298.20557, "y"=249.65573, "z"=0.9842166}, "UV"={"u"=0.0, "v"=0.0}, "Colour"=12517256}, "Alpha"=0.0, "Alpha Blending Enabled"=FALSE, "Colour"=9947756}, {"Vertex 1"={"Position"={"x"=497.92285, "y"=125.52894, "z"=0.98443836}, "UV"={"u"=0.0, "v"=0.0}, "Colour"=12517256}, "Vertex 2"={"Position"={"x"=492.5376, "y"=114.58211, "z"=0.98474693}, "UV"={"u"=0.0, "v"=0.0}, "Colour"=12517256}, "Vertex 3"={"Position"={"x"=448.60507, "y"=110.63302, "z"=0.984421}, "UV"={"u"=0.0, "v"=0.0}, "Colour"=12517256}, "Alpha"=0.0, "Alpha Blending Enabled"=FALSE, "Colour"=1581073}, {"Vertex 1"={"Position"={"x"=353.04034, "y"=323.3558, "z"=0.9846115}, "UV"={"u"=0.0, "v"=0.0}, "Colour"=12517256}, "Vertex 2"={"Position"={"x"=350.56738, "y"=298.80087, "z"=0.9843252}, "UV"={"u"=0.0, "v"=0.0}, "Colour"=12517256}, "Vertex 3"={"Position"={"x"=305.9204, "y"=298.8263, "z"=0.9846586}, "UV"={"u"=0.0, "v"=0.0}, "Colour"=12517256}, "Alpha"=0.0, "Alpha Blending Enabled"=FALSE, "Colour"=11199866}, {"Vertex 1"={"Position"={"x"=501.79443, "y"=249.65573, "z"=0.9842166}, "UV"={"u"=0.0, "v"=0.0}, "Colour"=12517256}, "Vertex 2"={"Position"={"x"=498.2464, "y"=274.33585, "z"=0.9844198}, "UV"={"u"=0.0, "v"=0.0}, "Colour"=12517256}, "Vertex 3"={"Position"={"x"=537.67664, "y"=275.21597, "z"=0.9849558}, "UV"={"u"=0.0, "v"=0.0}, "Colour"=12517256}, "Alpha"=0.0, "Alpha Blending Enabled"=FALSE, "Colour"=10343024}, {"Vertex 1"={"Position"={"x"=297.47644, "y"=139.52065, "z"=0.9841747}, "UV"={"u"=0.0, "v"=0.0}, "Colour"=12517256}, "Vertex 2"={"Position"={"x"=302.07715, "y"=125.52894, "z"=0.98443836}, "UV"={"u"=0.0, "v"=0.0}, "Colour"=12517256}, "Vertex 3"={"Position"={"x"=262.76135, "y"=131.49307, "z"=0.984972}, "UV"={"u"=0.0, "v"=0.0}, "Colour"=12517256}, "Alpha"=0.0, "Alpha Blending Enabled"=FALSE, "Colour"=2964512}, {"Vertex 1"={"Position"={"x"=547.78455, 
